vi "save_file.vi"(5 "write OME header?":bool=TRUE, 7 "path":path, 8 "error in (no error)":errorcluster, 10 "ImageCollection in":refnum<class "ImageCollection.lvclass">, 11 "DataCollectionDL090215 in":refnum<class "DataCollectionDL090215.lvclass">) -> (0 "error out":errorcluster, 3 "DataCollectionDL090215 out":refnum<class "DataCollectionDL090215.lvclass">)   [LabVIEW 2010, in "DataCollectionDL090215.lvclass"]
uses:
  DataCollectionDL090215.lvclass
  common/classes/ImageCollection/ImageCollection/dimension_order_enum.ctl
  common/classes/ImageCollection/ImageCollection/OME_parameters_cluster.ctl
  common/classes/ImageCollection/ImageCollection/ImageCollection.lvclass
  common/classes/XMLElement/XMLElement/XMLElement.lvclass
  common/classes/ErrorController/ErrorController/ErrorController.lvclass
  common/classes/Image/Image/target_format_enum.ctl
  common/classes/ImageCollection/ImageCollection/saving_parameters_cluster.ctl
panel:
  out "time needed to create TIFF file [ms]":u32
  out "time needed to compile OME XML element [ms]":u32
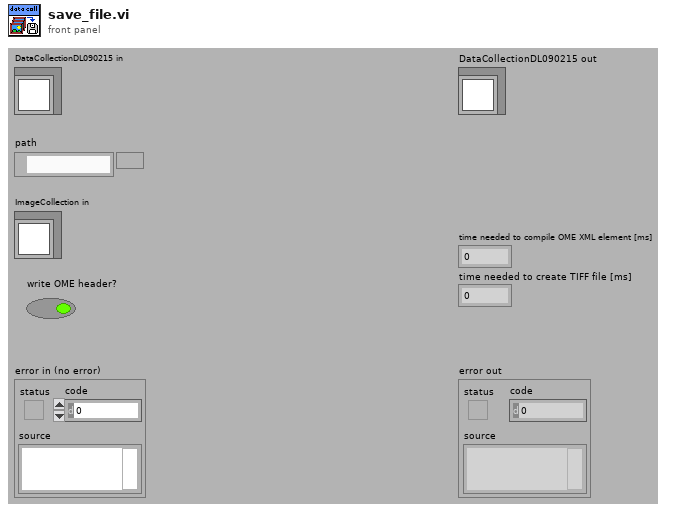
[diagram p1: front panel]
types:
  T1 = typedef "ImageCollection.lvclass/saving_parameters_cluster.ctl" = cluster{"write OME header?":bool, "save as list file?":bool, "force format?":T2, "multiplication factor":dbl, "offset":dbl}
  T2 = typedef "target_format_enum.ctl" = enum16{"don't force", "uint8", "uint16", "int16", "uint32", "int32", "single float"}
  T3 = typedef "dimension_order_enum.ctl" = enum16{"XYZCT", "XYZTC", "XYCTZ", "XYCZT", "XYTCZ", "XYTZC"}
  T4 = typedef "OME_parameters_cluster.ctl" = cluster{"image ID":string, "pixels ID":string, "dimension order":T3, "number of channels":i32}
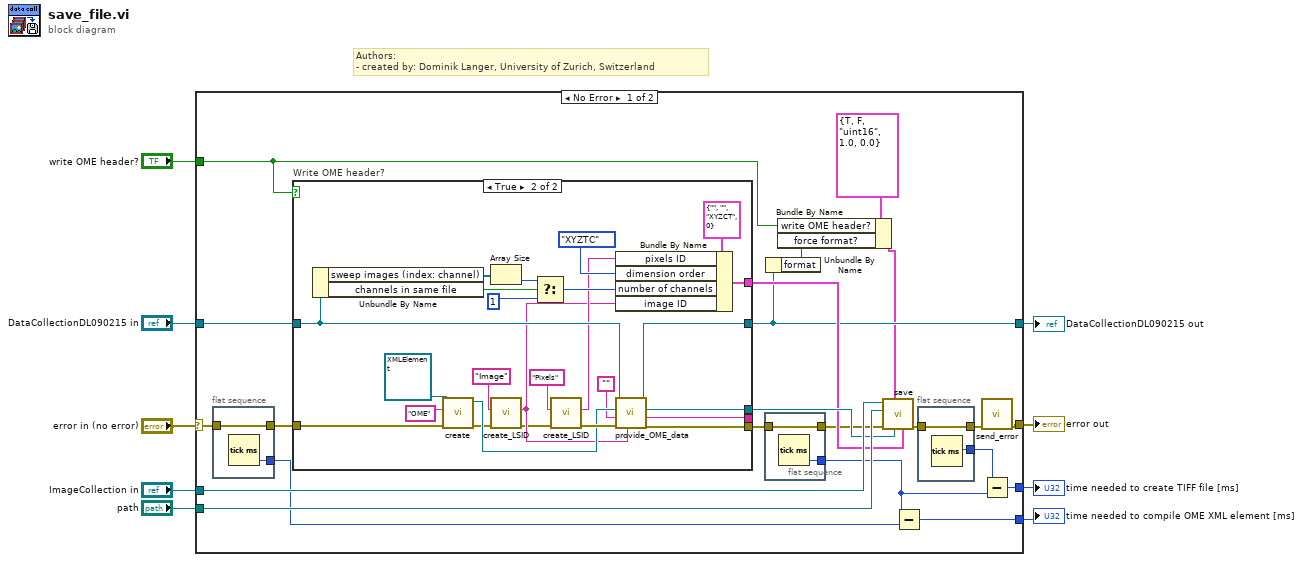
[diagram p0: block diagram]
diagram:
  # "Authors: \n- created by: Dominik Langer, University of Zurich, Switzerland"
  n1 = case shown="No Error" "error in (no error)" {
    selector: "error in (no error)" -> [w19 w66]
    tunnel: [w16 w66] -> w8
    tunnel: [w23 w65] -> w6
    tunnel: "DataCollectionDL090215 in" -> [w29 w65]
    tunnel: "path" -> [w31 _]
    tunnel: "ImageCollection in" -> [w30 _]
    tunnel: [w25 _] -> w3
    tunnel: [w17 _] -> w2
    tunnel: "write OME header?" -> [w11 _]
    frame No Error {
      n2 = flat-sequence {
        tunnel: [w33] -> w18
        tunnel: w19 -> [w33]
        tunnel: [w32] -> w10
        frame #0 {
          n3 = Tick Count (ms)() -> (millisecond timer value=w32:u32)
        }
      }
      n4 = case "Write OME header?" shown="True" w11 {
        tunnel: w29 -> [w36 w54]
        tunnel: [_ w52] -> w28
        tunnel: [_ w51] -> w27
        tunnel: [w37 w48] -> w22
        tunnel: w18 -> [w37 w47]
        tunnel: [w36 w49] -> w23
        tunnel: [_ w41] -> _
        frame False {
        }
        frame True {
          n5 = Unbundle By Name(w54) -> ("sweep images (index: channel)"=w56:refnum<class "ImageCollection.lvclass">[], "channels in same file"=w55:bool)
          n6 = call "create.vi"("error in (no error)"=w47, "name"="OME", "XMLElement in"=refnum<class "XMLElement.lvclass"> refnum ("XMLElement.lvclass")) -> ("error out"=w38:errorcluster, "XMLElement out"=w46:refnum<class "XMLElement.lvclass">)  [unwired: 7 in]
          n7 = Array Size(array=w56) -> (size(s)=w40:i32)
          n8 = call "create_LSID.vi"("error in (no error)"=w38, "namespace"="Image") -> ("error out"=w39:errorcluster, "LSID"=w43:string)  [unwired: 8 in]
          n9 = Select(t=w40, s=w55, f=1) -> (s? t:f=w60:i32)
          n10 = call "create_LSID.vi"("error in (no error)"=w39, "namespace"="Pixels") -> ("error out"=w50:errorcluster, "LSID"=w53:string)  [unwired: 8 in]
          n11 = Bundle By Name(cluster=T4 {"image ID"="", "pixels ID"="", "dimension order"=enum."XYZCT", "number of channels"=0} ("OME parameters"), "pixels ID"=w53, "dimension order"=dimension_order_enum."XYZTC", "number of channels"=w60, "image ID"=w43) -> (w51:T4)
          n12 = call-dynamic "provide_OME_data.vi"("image ID"=w43, "error in (no error)"=w50, "structuredAttribute string in"="", "OME element in"=w46, "DataCollectionDL091104Scaffold in"=w54) -> ("error out"=w48:errorcluster, "structuredAttribute string out"=w41:string, "OME element out"=w52:refnum<class "XMLElement.lvclass">, "DataCollectionDL091104Scaffold out"=w49:refnum<class "DataCollectionDL090215.lvclass">)  [unwired: 3 in]
        }
      }
      n13 = flat-sequence {
        tunnel: [w35] -> w21
        tunnel: w22 -> [w35]
        tunnel: [w34] -> w20
        frame #0 {
          n14 = Tick Count (ms)() -> (millisecond timer value=w34:u32)
        }
      }
      n15 = Unbundle By Name(w23) -> ("format"=w13:T2)
      n16 = Bundle By Name(cluster=T1 {"write OME header?"=TRUE, "save as list file?"=FALSE, "force format?"=enum."uint16", "multiplication factor"=1.0, "offset"=0.0} ("saving parameters"), "write OME header?"=w11, "force format?"=w13) -> (w12:T1)
      n17 = call "save.vi"("OME parameters"=w27, "OME XMLElement"=w28, "saving parameters"=w12, "error in (no error)"=w21, "path"=w31, "ImageCollection in"=w30) -> ("error out"=w26:errorcluster)  [unwired: 1 in, 4 out]
      n18 = Subtract(x=w20, y=w10) -> (x-y=w17:u32)
      n19 = flat-sequence {
        tunnel: [w64] -> w15
        tunnel: w26 -> [w64]
        tunnel: [w63] -> w24
        frame #0 {
          n20 = Tick Count (ms)() -> (millisecond timer value=w63:u32)
        }
      }
      n21 = call "send_error.vi"("error in (no error)"=w15) -> ("error out"=w16:errorcluster)  [unwired: 10 in]
      n22 = Subtract(x=w24, y=w20) -> (x-y=w25:u32)
    }
    frame Error {
    }
  }
  "error out" <- w8
  "DataCollectionDL090215 out" <- w6
  "time needed to compile OME XML element [ms]" <- w2
  "time needed to create TIFF file [ms]" <- w3
